vi "Test Ramp Field.vi"(6 "Axis":T1=enum."Y", 8 "error in (no error)":errorcluster, 9 "Target Field Rate (T/min)":dbl=0.05 format="%#_13g", 10 "Target Field (T)":dbl=0.05 format="%#_13g", 11 "Instrument.OxfordVRM in":refnum<class "Instrument.OxfordVRM.lvclass">) -> (0 "error out":errorcluster, 3 "Instrument.OxfordVRM out":refnum<class "Instrument.OxfordVRM.lvclass">)   [LabVIEW 2019, in "Instrument.OxfordVRM.lvclass"]
uses:
  Instrument.OxfordVRM.lvclass
  <vilib>/addons/_JKI Toolkits/Caraya/classes/Test/Test.lvclass
  <vilib>/addons/_JKI Toolkits/Caraya/classes/Assert/Assert.lvclass
  <vilib>/addons/_JKI Toolkits/Caraya/classes/Assert/Assert Not Error.vi
  <vilib>/addons/_JKI Toolkits/Caraya/classes/Assert/Assert Almost Equal_Float.vi
  <vilib>/addons/_JKI Toolkits/Caraya/classes/Assert/Assert Equal Value and Type_Variant.vi
  <userlib>/LevyLab/Instrument Framework/Instrument Types/Cryostat/Typedefs/Magnet Axis--Enum.ctl
  <userlib>/LevyLab/Instrument Framework/Instrument Types/Cryostat/Instrument.Cryostat.lvclass
panel:
  out "Power Supply Field (T)":dbl
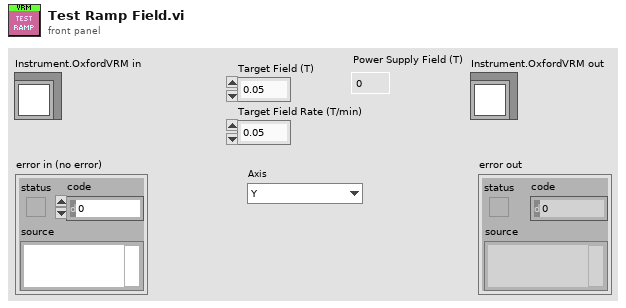
[diagram p1: front panel]
types:
  T1 = typedef "Instrument.Cryostat.lvclass/Magnet Axis--Enum.ctl" = enum16{"X", "Y", "Z"}
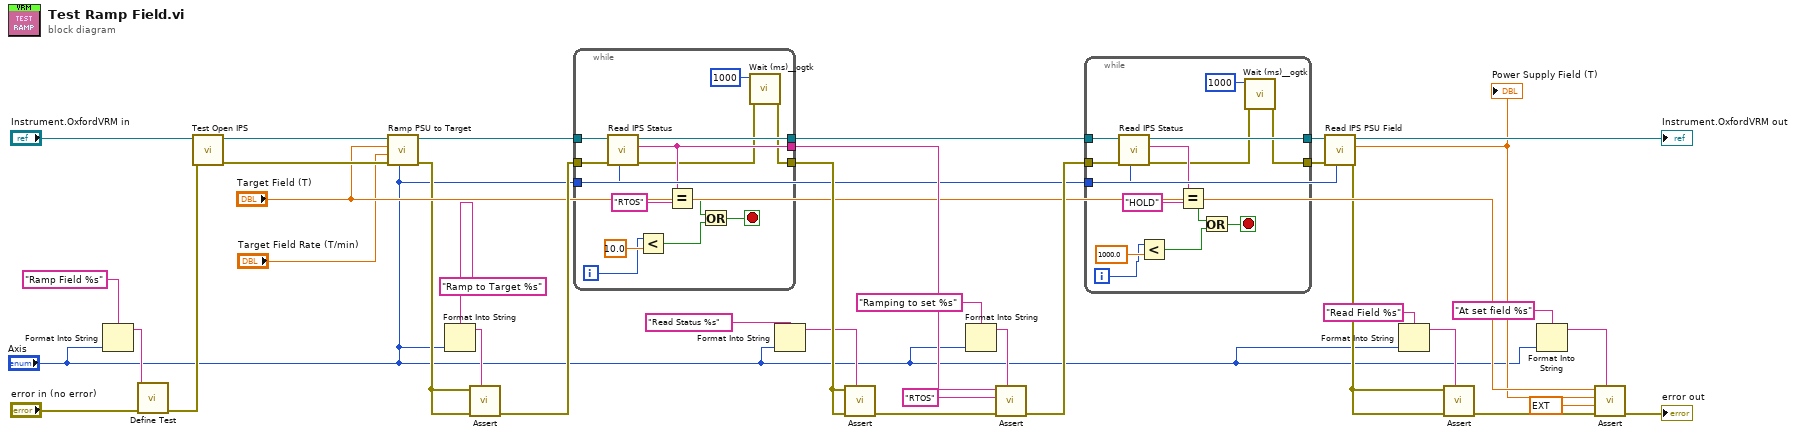
[diagram p0: block diagram]
diagram:
  n1 = Format Into String(format string="Ramp Field %s" ("Label (VI Title)"), "Axis") -> (resulting string=w12:string)  [unwired: 2 in, 1 out]
  n2 = call <vilib>:"Define Test.vi"("error in (no error)"="error in (no error)", "Label (VI Title)"=w12) -> ("error out"=w16:errorcluster)  [unwired: 8 in, 1 out]
  n3 = call "Test Open IPS.vi"("error in (no error)"=w16, "Instrument.OxfordVRM in"="Instrument.OxfordVRM in") -> ("error out"=w22:errorcluster, "Instrument.OxfordVRM out"=w23:refnum<class "Instrument.OxfordVRM.lvclass">)  [unwired: 8 in]
  n4 = call "Ramp PSU to Target.vi"("Axis"="Axis", "error in (no error)"=w22, "Target Rate (T/min)"="Target Field Rate (T/min)", "Target Field (T)"="Target Field (T)", "Instrument.OxfordVRM in"=w23) -> ("error out"=w17:errorcluster, "Instrument.OxfordVRM out"=w34:refnum<class "Instrument.OxfordVRM.lvclass">)  [unwired: 5 in]
  n5 = Format Into String(format string="Ramp to Target %s" ("Label"), "Axis") -> (resulting string=w10:string)  [unwired: 2 in, 1 out]
  n6 = call-poly <vilib>:"Assert.vi"("Label"=w10, "error in (no error)"=w17, "Not Error?"=w17) -> ("error out"=w35:errorcluster)  [unwired: 7 in, 1 out]
  n7 = while {
    tunnel: [w48] -> w31
    tunnel: w34 -> [w50]
    tunnel: [w49] -> w18
    tunnel: w35 -> [w51]
    tunnel: [w39] -> w33
    tunnel: "Axis" -> [w38]
    i -> [w44]
    stop <- w43 stop-if-true
    n8 = call "Read IPS Status.vi"("Axis"=w38, "error in (no error)"=w51, "Instrument.OxfordVRM in"=w50) -> ("error out"=w40:errorcluster, "Status"=w48:string, "Instrument.OxfordVRM out"=w49:refnum<class "Instrument.OxfordVRM.lvclass">)  [unwired: 6 in]
    n9 = Less?(x=w44, y=10.0) -> (x < y?=w41:bool)
    n10 = Equal?(x=w48, y="RTOS") -> (x = y?=w42:bool)
    n11 = Or(x=w42, y=w41) -> (x .or. y?=w43:bool)
    n12 = call <userlib>:"Wait (ms)__ogtk.vi"("error in (no error)"=w40, "milliseconds to wait"=u32 1000) -> ("error out"=w39:errorcluster)  [unwired: 8 in, 1 out]
  }
  n13 = Format Into String(format string="Read Status %s" ("Label"), "Axis") -> (resulting string=w9:string)  [unwired: 2 in, 1 out]
  n14 = call-poly <vilib>:"Assert.vi"("Label"=w9, "error in (no error)"=w33, "Not Error?"=w33) -> ("error out"=w32:errorcluster)  [unwired: 7 in, 1 out]
  n15 = Format Into String(format string="Ramping to set %s" ("Label"), "Axis") -> (resulting string=w7:string)  [unwired: 2 in, 1 out]
  n16 = call-poly <vilib>:"Assert.vi"("Label"=w7, "error in (no error)"=w32, "Y"="RTOS", "X"=w31) -> ("error out"=w25:errorcluster)  [unwired: 6 in, 1 out]
  n17 = while {
    tunnel: w18 -> [w64]
    tunnel: [w63] -> w19
    tunnel: w25 -> [w65]
    tunnel: [w53] -> w24
    tunnel: "Axis" -> [w52]
    i -> [w55]
    stop <- w56 stop-if-true
    n18 = call "Read IPS Status.vi"("Axis"=w52, "error in (no error)"=w65, "Instrument.OxfordVRM in"=w64) -> ("error out"=w54:errorcluster, "Status"=w62:string, "Instrument.OxfordVRM out"=w63:refnum<class "Instrument.OxfordVRM.lvclass">)  [unwired: 6 in]
    n19 = Less?(x=w55, y=1000.0) -> (x < y?=w58:bool)
    n20 = Equal?(x=w62, y="HOLD") -> (x = y?=w57:bool)
    n21 = Or(x=w57, y=w58) -> (x .or. y?=w56:bool)
    n22 = call <userlib>:"Wait (ms)__ogtk.vi"("error in (no error)"=w54, "milliseconds to wait"=u32 1000) -> ("error out"=w53:errorcluster)  [unwired: 8 in, 1 out]
  }
  n23 = call "Read IPS PSU Field.vi"("Axis"="Axis", "error in (no error)"=w24, "Instrument.OxfordVRM in"=w19) -> ("error out"=w14:errorcluster, "Power Supply Field (T)"=w15:dbl, "Instrument.OxfordVRM out"=→"Instrument.OxfordVRM out":refnum<class "Instrument.OxfordVRM.lvclass">)  [unwired: 6 in]
  "Power Supply Field (T)" <- w15
  n24 = Format Into String(format string="Read Field %s" ("Label"), "Axis") -> (resulting string=w5:string)  [unwired: 2 in, 1 out]
  n25 = call-poly <vilib>:"Assert.vi"("Label"=w5, "error in (no error)"=w14, "Not Error?"=w14) -> ("error out"=w29:errorcluster)  [unwired: 7 in, 1 out]
  n26 = Format Into String(format string="At set field %s" ("Label"), "Axis") -> (resulting string=w2:string)  [unwired: 2 in, 1 out]
  n27 = call-poly <vilib>:"Assert.vi"("Label"=w2, "error in (no error)"=w29, "Tolerance"=ext 0.00099999999999999999996, "Y"=w15, "X"="Target Field (T)") -> ("error out"=→"error out":errorcluster)  [unwired: 5 in, 1 out]
